vi "dump.vi"(8 "error in (no error)":errorcluster, 10 "indent":T1, 11 "FloatType in":refnum<class "FloatType.lvclass">) -> (0 "error out":errorcluster, 2 "mlir":string, 3 "FloatType out":refnum<class "FloatType.lvclass">)   [LabVIEW 2020, in "mlir.lvlib" / "FloatType.lvclass"]
uses:
  FloatType.lvclass
  Node/indent.ctl
  FloatType.lvclass/FloatType.ctl
  mlir.lvlib
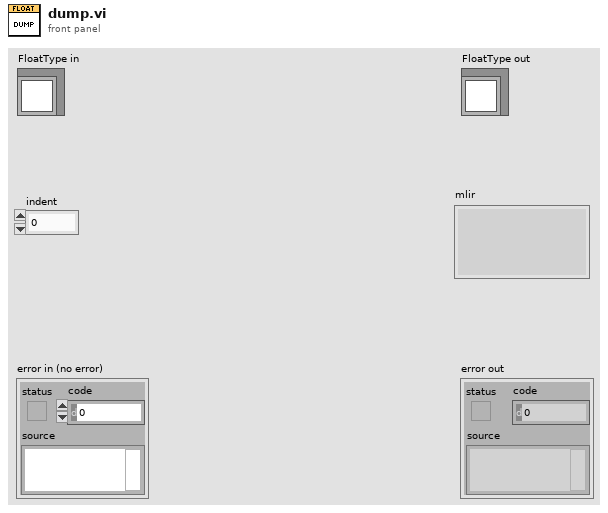
[diagram p1: front panel]
types:
  T1 = typedef "mlir.lvlib/indent.ctl" = u32
  T2 = typedef "mlir.lvlib/FloatType.lvclass/FloatTypeEnum.ctl" = enum16{"f16", "bf16", "f32", "f64"}
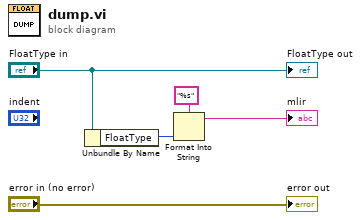
[diagram p0: block diagram]
diagram:
  n1 = Unbundle By Name("FloatType in") -> ("FloatType"=w3:T2)
  n2 = Format Into String(format string="%s", w3) -> (resulting string=→"mlir":string)  [unwired: 2 in, 1 out]
  "error out" <- "error in (no error)"
  "FloatType out" <- "FloatType in"
